vi "Trim String.vi"(11 "String":string) -> (3 "trimmed string":string)   [LabVIEW 2011, in "Tinkerforge.lvlib"]
doc: "This VI trimms all \"\\00\" at the end of the string."
uses:
  Tinkerforge.lvlib
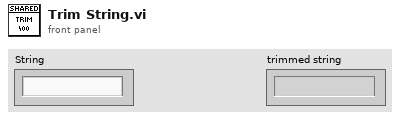
[diagram p1: front panel]
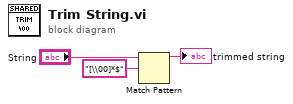
[diagram p0: block diagram]
diagram:
  n1 = Match Pattern(string="String", regular expression="[\\00]*$") -> (before substring=→"trimmed string":string)  [unwired: 1 in, 3 out]
